vi "Build Data Table for Simplestat.vi"(10 "Table":T1[](array[typedef]), 11 "Frequency Array":dbl[](array[numeric])) -> (2 "All Data by Frequency":cluster{"Array":dbl[]}[](array[cluster]), 3 "Channel Data":dbl[][](array[numeric]))   [LabVIEW 2011]
uses:
  CGI SimpleStat Results.ctl
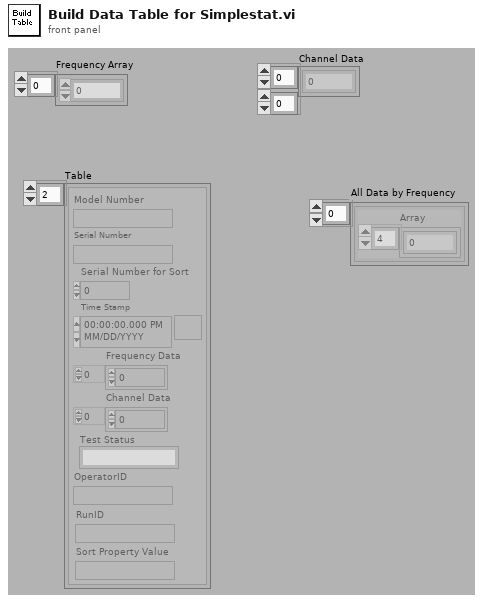
[diagram p1: front panel]
types:
  T1 = typedef "CGI SimpleStat Results.ctl" = cluster{"Model Number":string, "Serial Number for Sort":i32, "Serial Number":string, "Time Stamp":timestamp, "Channel Data":dbl[], "Test Status":string, "OperatorID":string, "Frequency Data":dbl[], "RunID":string, "Sort Property Value":string}
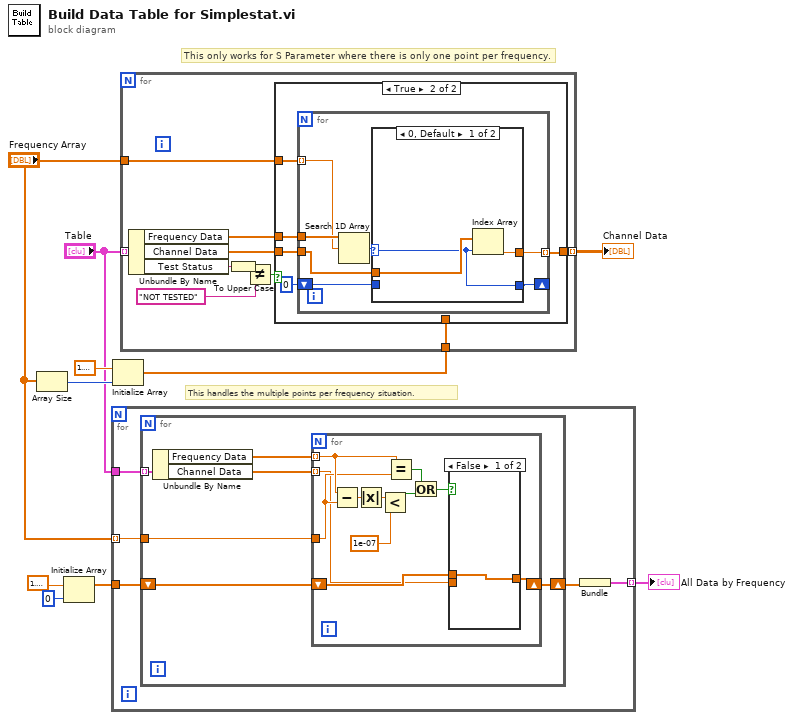
[diagram p0: block diagram]
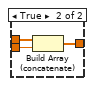
[diagram p2: hidden frame]
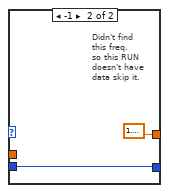
[diagram p4: hidden frame]
diagram:
  # "This only works for S Parameter where there is only one point per frequency."
  # "This handles the multiple points per frequency situation."
  n1 = Array Size(array="Frequency Array") -> (size(s)=w8:i32)
  n2 = Initialize Array(1.1447298858494002, 0 ("dimension size")) -> (w1:dbl[])
  n3 = for {
    tunnel: "Table" -> [w15]
    tunnel: "Frequency Array" -> [w14] mode=indexing
    tunnel: [w12] -> w4 mode=indexing
    tunnel: w1 -> [w11]
    n4 = for {
      tunnel: w15 -> [w21] mode=indexing
      tunnel: w14 -> [w19]
      shift-right: [w17] -> w13
      shift-left: w11 -> [w16]
      n5 = Unbundle By Name(w21) -> ("Frequency Data"=w20:dbl[], "Channel Data"=w18:dbl[])
      n6 = for {
        tunnel: w20 -> [w27] mode=indexing
        shift-right: [w22] -> w17
        shift-left: w16 -> [w24]
        tunnel: w19 -> [w26]
        tunnel: w18 -> [w23] mode=indexing
        n7 = Subtract(x=w27, y=w26) -> (x-y=w29:dbl)
        n8 = Absolute Value(x=w29) -> (abs(x)=w28:dbl)
        n9 = Less?(x=w28, y=1e-07) -> (x < y?=w30:bool)
        n10 = Equal?(x=w27, y=w26) -> (x = y?=w32:bool)
        n11 = Or(x=w32, y=w30) -> (x .or. y?=w25:bool)
        n12 = case shown="False" w25 {
          tunnel: w24 -> [w33 w36]
          tunnel: w23 -> [_ w35]
          tunnel: [w33 w34] -> w22
          frame False {
          }
          frame True {
            n13 = Build Array (concatenate)(w36, w35) -> (w34:dbl[])
          }
        }
      }
    }
    n14 = Bundle(w13) -> (w12:cluster{dbl[]})  [unwired: 1 in]
  }
  "All Data by Frequency" <- w4
  n15 = Initialize Array(1.1447298858494002, w8) -> (w9:dbl[])
  n16 = for {
    tunnel: "Table" -> [w46] mode=indexing
    tunnel: [w42] -> w10 mode=indexing
    tunnel: w9 -> [w43]
    tunnel: "Frequency Array" -> [w41]
    n17 = Unbundle By Name(w46) -> ("Frequency Data"=w40:dbl[], "Channel Data"=w39:dbl[], "Test Status"=w45:string)
    n18 = To Upper Case(1:w45) -> (0:w37:string)
    n19 = Not Equal?(x=w37, y="NOT TESTED") -> (x != y?=w44:bool)
    n20 = case shown="True" w44 {
      tunnel: w43 -> [w47 _]
      tunnel: [w47 w50] -> w42
      tunnel: w41 -> [_ w52]
      tunnel: w40 -> [_ w51]
      tunnel: w39 -> [_ w49]
      frame False {
        # "This column should be all LNPI"
      }
      frame True {
        n21 = for {
          tunnel: w52 -> [w58] mode=indexing
          tunnel: w51 -> [w59]
          tunnel: [w56] -> w50 mode=indexing
          tunnel: w49 -> [w55]
          shift-right: [w54] -> _
          shift-left: 0 ("index of element") -> [w53]
          n22 = Search 1D Array(1D array=w59, element=w58) -> (index of element=w57:i32)  [unwired: 1 out]
          n23 = case shown="0, Default" w57 {
            selector: w57 -> [w60 _]
            tunnel: [w61 1.1447298858494002] -> w56
            tunnel: w55 -> [w62 _]
            tunnel: [w60 w64] -> w54
            tunnel: w53 -> [_ w64]
            frame 0, Default {
              n24 = Index Array(array=w62, index=w60) -> (element=w61:dbl)
            }
            frame -1 {
              # "Didn't find \nthis freq.\nso this RUN\ndoesn't have\ndata skip it."
            }
          }
        }
      }
    }
  }
  "Channel Data" <- w10
